vi "Read Method.vi"(8 "error in (no error)":errorcluster, 11 "Width Method in":refnum<class "Width Method.lvclass">) -> (0 "error out":errorcluster, 2 "Width in":T1, 3 "Width Method out":refnum<class "Width Method.lvclass">)   [LabVIEW 2014, in "Width Method.lvclass"]
uses:
  Width Method.lvclass
  Utility/Width Method.ctl
  Width Method.lvclass/Width Method.ctl
  Utility/POLARIS Vision utility.lvlib
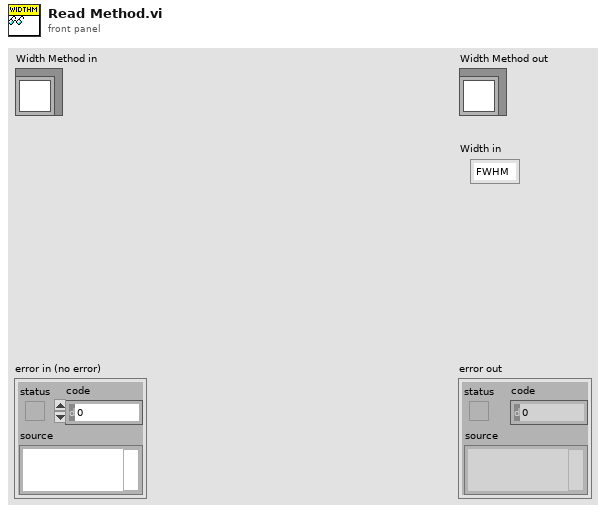
[diagram p1: front panel]
types:
  T1 = typedef "POLARIS Vision utility.lvlib/Width Method.ctl" = enum16{"FWHM", "1/e", "1/e^2", "80%", "90%"}
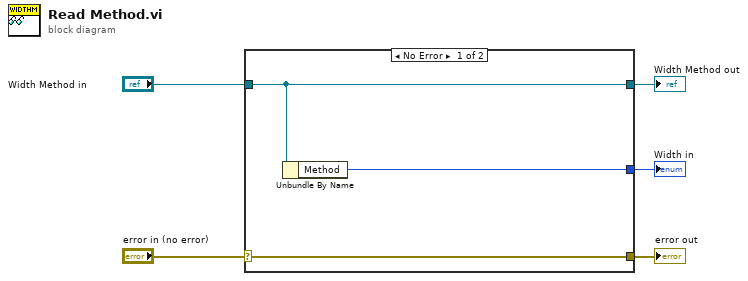
[diagram p0: block diagram]
diagram:
  n1 = case shown="No Error" "error in (no error)" {
    selector: "error in (no error)" -> [w8 w9]
    tunnel: [w8 w9] -> w4
    tunnel: [w7 w10] -> w2
    tunnel: "Width Method in" -> [w7 w10]
    tunnel: [w6 _] -> w1
    frame No Error {
      n2 = Unbundle By Name(w7) -> ("Method"=w6:T1)
    }
    frame Error {
    }
  }
  "error out" <- w4
  "Width Method out" <- w2
  "Width in" <- w1
